vi "Add Character.vi"(8 "error in (no error)":errorcluster, 9 "Input Array":u16[](array[numeric]), 11 "Character":string) -> (0 "error out":errorcluster, 1 "Output Array":u16[](array[numeric]))   [LabVIEW 2015]
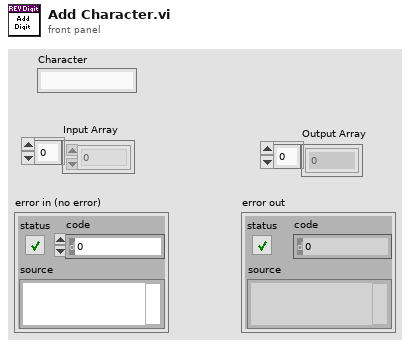
[diagram p1: front panel]
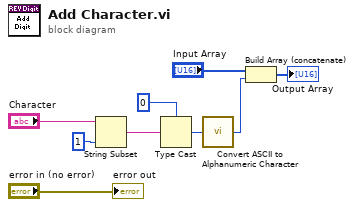
[diagram p0: block diagram]
diagram:
  n1 = String Subset(string="Character", length (rest)=1 ("length (rest)")) -> (substring=w4:string)  [unwired: 1 in]
  n2 = Type Cast(type=u8 0 ("length (rest)"), x=w4) -> (*(type *) &x=w2:u8)
  n3 = call "Convert ASCII to Alphanumeric Character.vi"("ASCII Value"=w2) -> ("Alphanumeric Character Value"=w6:u16)
  n4 = Build Array (concatenate)("Input Array", w6) -> (→"Output Array":u16[])
  "error out" <- "error in (no error)"
